vi "populate_pointCollection.vi"(7 "calibration":dbl[unit][](array[numeric])=[1e-06, 1e-06, 1e-06], 8 "error in (no error)":errorcluster, 10 "ROI:ROIs":T1(array[cluster]), 11 "PointCollection.lvclass in":refnum<class "PointCollection.lvclass">) -> (0 "error out":errorcluster, 3 "PointCollection.lvclass out":refnum<class "PointCollection.lvclass">)   [LabVIEW 2010]
uses:
  common/classes/PointCollection/PointCollection/PointCollection.lvclass
  common/classes/PointCollection/PointCollection/mode_enum.ctl
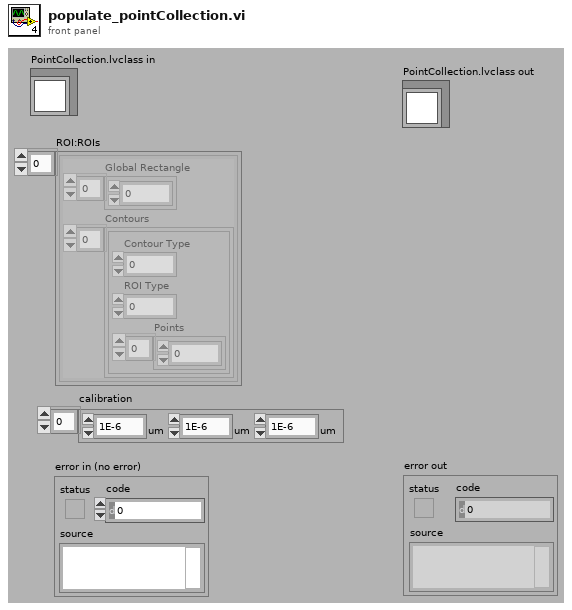
[diagram p1: front panel]
types:
  T1 = cluster{"Global Rectangle":i32[], "Contours":cluster{"Contour Type":u32, "ROI Type":u32, "Points":i32[]}[]}[]
  T2 = typedef "PointCollection.lvclass/mode_enum.ctl" = enum16{"points first", "dimensions first"}
  T3 = cluster{"Contour Type":u32, "ROI Type":u32, "Points":i32[]}[]
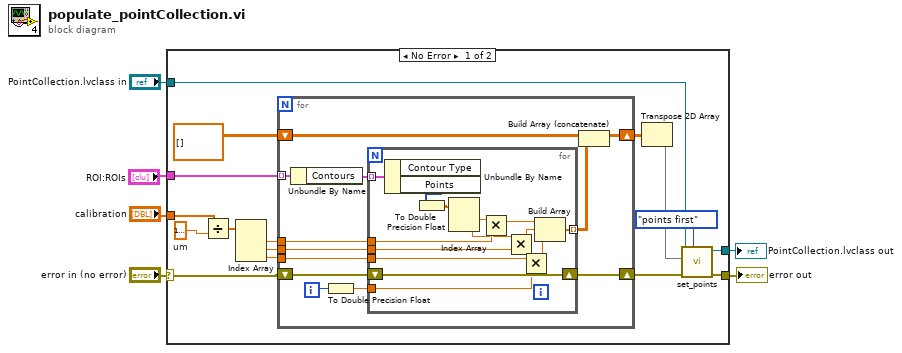
[diagram p0: block diagram]
diagram:
  n1 = case shown="No Error" "error in (no error)" {
    selector: "error in (no error)" -> [w22 w50]
    tunnel: "ROI:ROIs" -> [w21 _]
    tunnel: [w16 w50] -> w5
    tunnel: "calibration" -> [w19 _]
    tunnel: [w15 w49] -> w4
    tunnel: "PointCollection.lvclass in" -> [w14 w49]
    frame No Error {
      w20 = dbl[unit] 1e-06  # um
      n2 = Divide(x=w19, y=w20) -> (x/y=w11:dbl[])
      n3 = Index Array(array=w11) -> (element #1=w10:dbl, element #2=w9:dbl, element #3=w8:dbl)  [unwired: 3 in]
      n4 = for {
        tunnel: w21 -> [w34] mode=indexing
        shift-right: [w31] -> w17
        shift-left: w22 -> [w33]
        shift-right: [w28] -> w13
        shift-left: dbl[][] [] -> [w27]
        tunnel: w8 -> [w30]
        tunnel: w10 -> [w24]
        tunnel: w9 -> [w23]
        i -> [w26]
        n5 = Unbundle By Name(w34) -> ("Contours"=w32:T3)
        n6 = To Double Precision Float(number=w26) -> (double precision float=w25:dbl)
        n7 = for {
          shift-right: [w48] -> w31
          shift-left: w33 -> [w48]
          tunnel: w32 -> [w47] mode=indexing
          tunnel: [w45] -> w29 mode=indexing
          tunnel: w30 -> [w44]
          tunnel: w25 -> [w43]
          tunnel: w24 -> [w39]
          tunnel: w23 -> [w35]
          n8 = Unbundle By Name(w47) -> ("Points"=w42:i32[])  [unwired: 1 out]
          n9 = To Double Precision Float(number=w42) -> (double precision float=w41:dbl[])
          n10 = Index Array(array=w41) -> (element #1=w40:dbl, element #2=w37:dbl)  [unwired: 2 in]
          n11 = Multiply(x=w40, y=w39) -> (x*y=w38:dbl)
          n12 = Multiply(x=w37, y=w35) -> (x*y=w36:dbl)
          n13 = Multiply(x=w44, y=w43) -> (x*y=w46:dbl)
          n14 = Build Array(w38, w36, w46) -> (w45:dbl[])
        }
        n15 = Build Array (concatenate)(w27, w29) -> (w28:dbl[][])
      }
      n16 = Transpose 2D Array(2D array=w13) -> (transposed array=w12:dbl[][])
      n17 = call "set_points.vi"("mode"=mode_enum."points first", "error in (no error)"=w17, "points (dimensions/points)"=w12, "PointCollection in"=w14) -> ("error out"=w16:errorcluster, "PointCollection out"=w15:refnum<class "PointCollection.lvclass">)  [unwired: 6 in]
    }
    frame Error {
    }
  }
  "error out" <- w5
  "PointCollection.lvclass out" <- w4
